vi "Seriell lesen.vi"(8 "Fehler (Eingang)":errorcluster caption="Fehler (Eingang, kein Fehler)", 11 "VISA resource name":refnum<visa-resource-name>) -> (0 "error out":errorcluster, 1 "bytes read":u32, 2 "read buffer":string, 3 "VISA resource name":refnum<visa-resource-name>)   [LabVIEW 2020, in "AK-Schnittstelle.lvlib" / "AK Seriell.lvlib"]
uses:
  AK Seriell/AK Seriell.lvlib
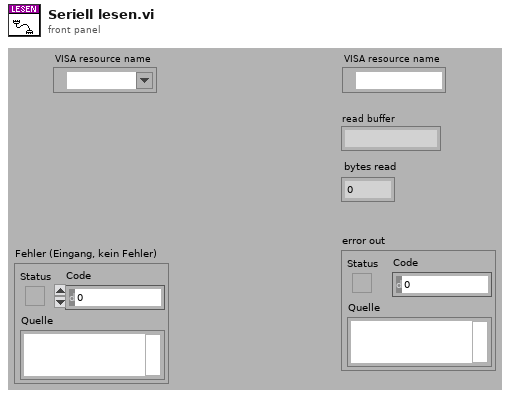
[diagram p1: front panel]
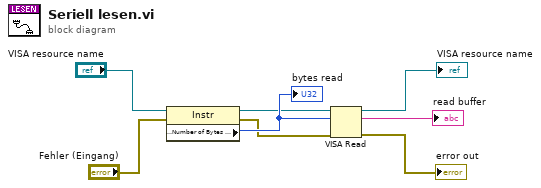
[diagram p0: block diagram]
diagram:
  n1 = property class="Instr"(reference="VISA resource name", error in="Fehler (Eingang)") -> (reference out=w5:refnum<visa-resource-name>, error out=w6:errorcluster, "Serial Settings:Number of Bytes at Serial Port"=w7:u32)
  "bytes read" <- w7
  n2 = VISA Read(VISA resource name=w5, byte count=w7, error in (no error)=w6) -> (VISA resource name out=→"VISA resource name":refnum<visa-resource-name>, read buffer=→"read buffer":string, error out=→"error out":errorcluster)  [unwired: 1 out]
